vi "niRFUtil FWK Active Channel Parser.vi"(0 "Active Channel":string, 5 "String Format":string[](array[string])=[""], 7 "Number of Channels":i32=1, 11 "error in (no error)":errorcluster, 12 "Mode":enum16{"Write", "Read"}(ring)) -> (6 "Channel Index":i32[](array[numeric]), 10 "Channel Name":string, 15 "error out":errorcluster)   [LabVIEW 2015, in "niRFUtil.lvlib"]
uses:
  niRFUtil.lvlib
  <vilib>/regexp/Match Regular Expression.xnode
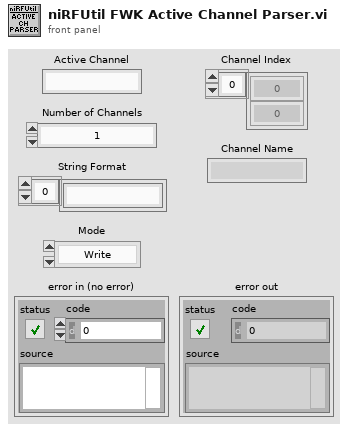
[diagram p1: front panel]
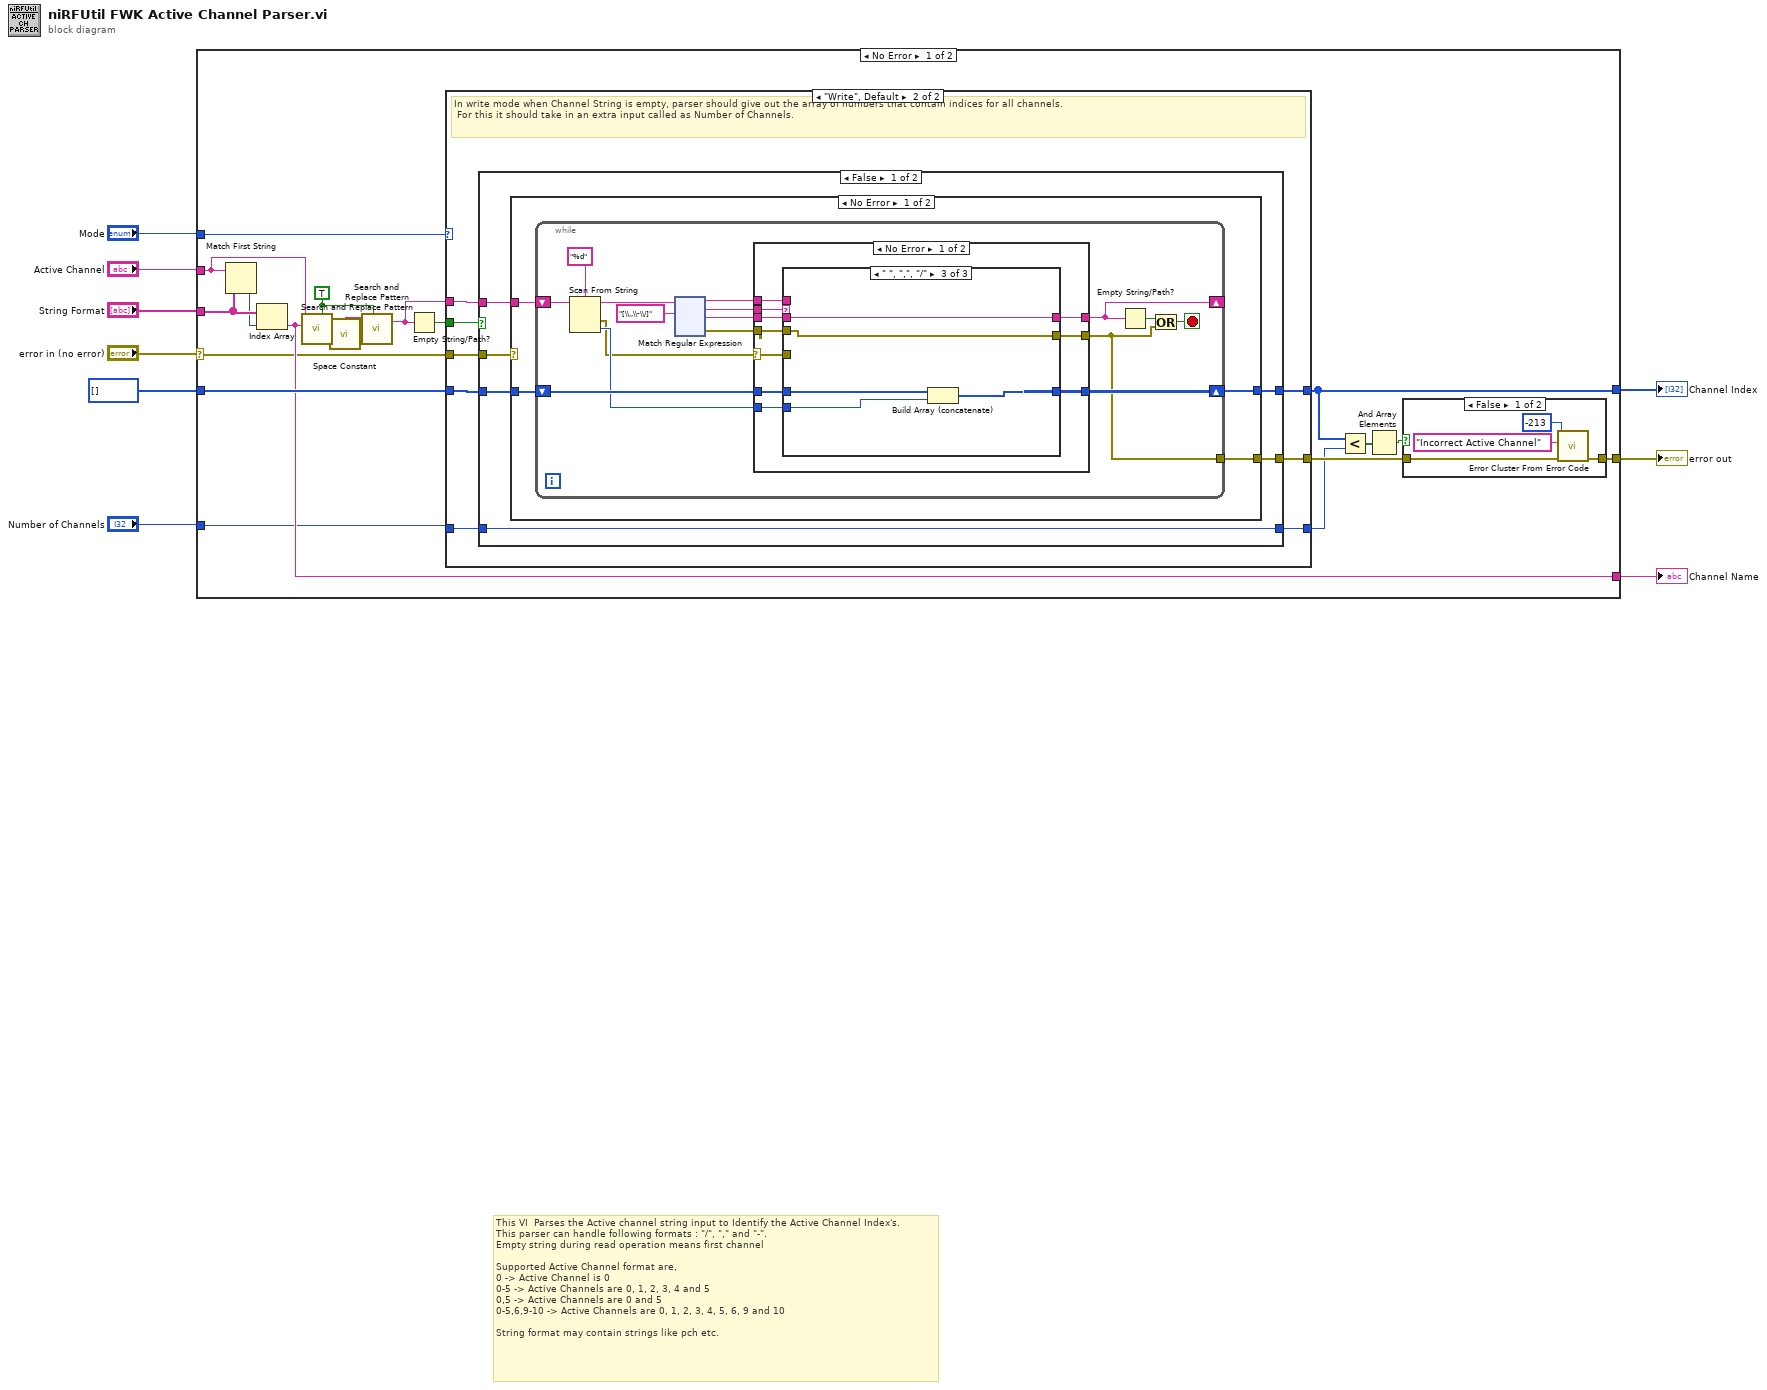
[diagram p0: block diagram]
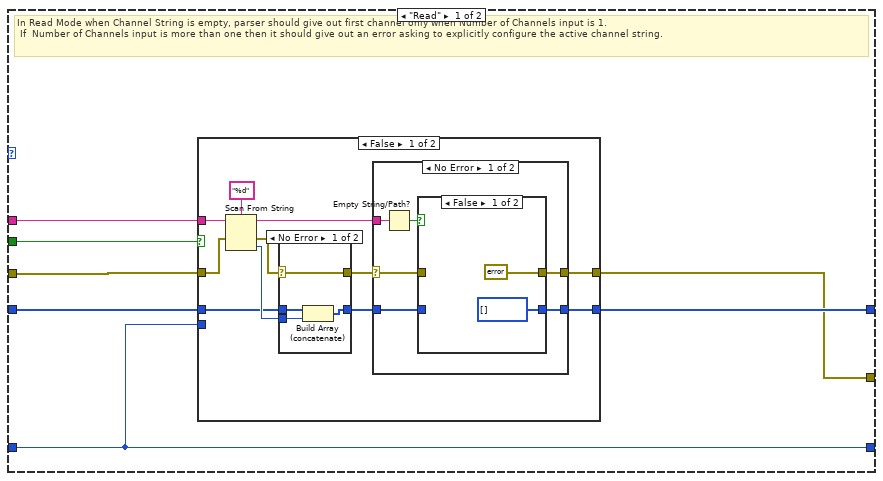
[diagram p3: hidden frame]
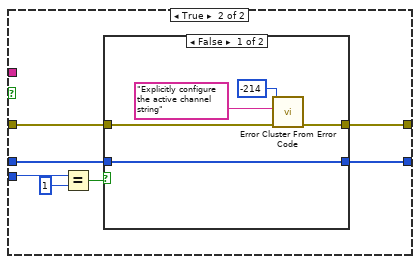
[diagram p7: hidden frame]
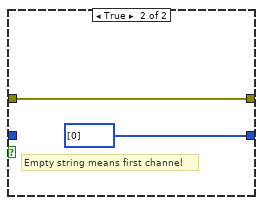
[diagram p8: hidden frame]
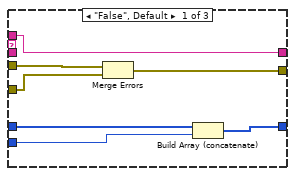
[diagram p9: hidden frame]
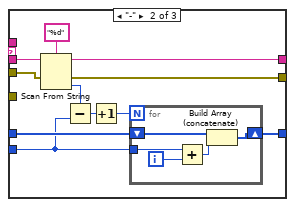
[diagram p10: hidden frame]
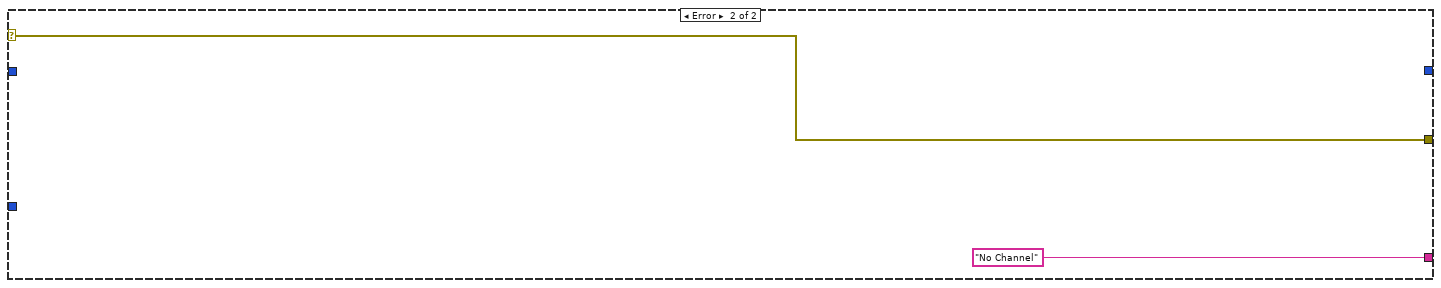
[diagram p14: hidden frame]
diagram:
  # "This VI  Parses the Active channel string input to Identify the Active Channel Index's.\nThis parser can handle following formats : \"/\", \",\" and \"-\".\nEmpty string during read operation means first channel\n\nSupported Active Channel format are,\n0 -> Active Channel is 0 \n0-5 -> Active Channels are 0, 1, 2, 3, 4 and 5\n0,5 -> Active Channels are 0 and 5\n0-5,6,9-10 -> Active Channels are 0, 1, 2, 3, 4, 5, 6, 9 and 10\n\nString format may contain strings like pch etc."
  n1 = case shown="No Error" "error in (no error)" {
    selector: "error in (no error)" -> [w22 w276]
    tunnel: i32[] [] -> [w27 _]
    tunnel: "Active Channel" -> [w24 _]
    tunnel: [w16 w276] -> w4
    tunnel: [w25 "No Channel"] -> w3
    tunnel: "Mode" -> [w23 _]
    tunnel: "String Format" -> [w21 _]
    tunnel: "Number of Channels" -> [w20 _]
    tunnel: [w15 _] -> w2
    frame No Error {
      w11 = TRUE ("replace all? (F)")
      n2 = Match First String(2:w21, 3:w24) -> (0:w14:i32)  [unwired: 1 out]
      n3 = Index Array(array=w21, index=w14) -> (element=w25:string)
      n4 = call <vilib>:"Search and Replace Pattern.vi"("string"=w24, "regular expression (\"\")"=w25, "replace all? (F)"=w11) -> ("result string"=w13:string)  [unwired: 2 in, 1 out]
      n5 = call <vilib>:"Space Constant.vi"() -> ("String"=w12:string)
      n6 = call <vilib>:"Search and Replace Pattern.vi"("string"=w13, "regular expression (\"\")"=w12, "replace all? (F)"=w11) -> ("result string"=w10:string)  [unwired: 2 in, 1 out]
      n7 = Empty String/Path?(string/path=w10) -> (empty?=w26:bool)
      n8 = case shown="\"Write\", Default" w23 {
        tunnel: w27 -> [w40 w91]
        tunnel: [w39 w90] -> w15
        tunnel: w26 -> [w38 w89]
        tunnel: [w37 w88] -> w28
        tunnel: w10 -> [w34 w87]
        tunnel: w22 -> [w36 w86]
        tunnel: w20 -> [w35 w85]
        tunnel: [w35 w84] -> w17
        frame "Read" {
          # "In Read Mode when Channel String is empty, parser should give out first channel only when Number of Channels input is 1.\n If  Number of Channels input is more than one then it should give out an error asking to explicitly configure the active channel string."
          n9 = case shown="False" w38 {
            tunnel: w40 -> [w46 w72]
            tunnel: [w51 w76] -> w39
            tunnel: w34 -> [w50 _]
            tunnel: [w42 w70] -> w37
            tunnel: w36 -> [w41 w71]
            tunnel: w35 -> [_ w75]
            frame False {
              n10 = Scan From String(format string="%d", input string=w50, error in=w41) -> (remaining string=w49:string, error out=w48:errorcluster, output 1=w47:i32)  [unwired: 2 in, 1 out]
              n11 = case shown="No Error" w48 {
                selector: w48 -> [w64 w68]
                tunnel: w47 -> [w65 _]
                tunnel: w46 -> [w67 w69]
                tunnel: [w66 w69] -> w45
                tunnel: [w64 w68] -> w43
                frame No Error {
                  n12 = Build Array (concatenate)(w67, w65) -> (w66:i32[])
                }
                frame Error {
                }
              }
              n13 = case shown="No Error" w43 {
                selector: w43 -> [w53 w62]
                tunnel: [w57 w63] -> w51
                tunnel: w49 -> [w56 _]
                tunnel: w45 -> [w55 w63]
                tunnel: [w54 w62] -> w42
                frame No Error {
                  n14 = Empty String/Path?(string/path=w56) -> (empty?=w52:bool)
                  n15 = case shown="False" w52 {
                    tunnel: [i32[] [] w61] -> w57
                    tunnel: w55 -> [_ w61]
                    tunnel: w53 -> [_ w60]
                    tunnel: [errorcluster {"status"=TRUE, "code"=-213, "source"="Incorrect Active Channel"} ("error IO") w60] -> w54
                    frame False {
                    }
                    frame True {
                    }
                  }
                }
                frame Error {
                }
              }
            }
            frame True {
              n16 = Equal?(x=w75, y=1) -> (x = y?=w73:bool)
              n17 = case shown="False" w73 {
                tunnel: [w81 i32[] [0]] -> w76
                tunnel: w72 -> [w81 _]
                tunnel: w71 -> [w77 w82]
                tunnel: [w78 w82] -> w70
                frame False {
                  n18 = call <vilib>:"Error Cluster From Error Code.vi"("error in (no error)"=w77, "error message (\"\")"="Explicitly configure the active channel string" ("error message (\"\")"), "error code (0)"=-214 ("code")) -> ("error out"=w78:errorcluster)  [unwired: 6 in]
                }
                frame True {
                  # "Empty string means first channel"
                }
              }
            }
          }
        }
        frame "Write", Default {
          # "In write mode when Channel String is empty, parser should give out the array of numbers that contain indices for all channels.\n For this it should take in an extra input called as Number of Channels."
          n19 = case shown="False" w89 {
            tunnel: w91 -> [w96 _]
            tunnel: [w97 w273] -> w90
            tunnel: w87 -> [w92 _]
            tunnel: [w94 w272] -> w88
            tunnel: w86 -> [w95 w272]
            tunnel: w85 -> [w93 w271]
            tunnel: [w93 w271] -> w84
            frame False {
              n20 = case shown="No Error" w95 {
                selector: w95 -> [_ w269]
                tunnel: [w101 w270] -> w97
                tunnel: w92 -> [w100 _]
                tunnel: w96 -> [w99 w270]
                tunnel: [w98 w269] -> w94
                frame No Error {
                  n21 = while {
                    shift-right: [w104] -> _
                    shift-left: w100 -> [w109]
                    shift-right: [w111] -> w101
                    shift-left: w99 -> [w115]
                    tunnel: [w103] -> w98
                    stop <- w112 stop-if-true
                    n22 = Scan From String(format string="%d", input string=w109) -> (remaining string=w108:string, error out=w105:errorcluster, output 1=w107:i32)  [unwired: 3 in, 1 out]
                    n23 = xnode "Match Regular Expression"("input string"=w108, "regular expression"="[\\,,\\-\\/]") -> ("before match"=w114:string, "whole match"=w117:string, "after match"=w116:string, "error out"=w106:errorcluster)  [unwired: 4 in, 1 out]
                    n24 = case shown="No Error" w105 {
                      selector: w105 -> [w118 _]
                      tunnel: w117 -> [w127 _]
                      tunnel: w116 -> [w126 w157]
                      tunnel: w115 -> [w125 w156]
                      tunnel: w114 -> [w124 _]
                      tunnel: [w123 w157] -> w104
                      tunnel: [w122 _] -> w103
                      tunnel: [w121 w156] -> w111
                      tunnel: w107 -> [w119 _]
                      tunnel: w106 -> [w120 _]
                      frame No Error {
                        n25 = case shown="\" \", \",\", \"/\"" w127 {
                          tunnel: w126 -> [_ w142 w153]
                          tunnel: [w128 w141 w153] -> w123
                          tunnel: [w132 w145 w155] -> w121
                          tunnel: w125 -> [w134 w144 w154]
                          tunnel: w124 -> [w128 _ _]
                          tunnel: [w129 w136 w151] -> w122
                          tunnel: w120 -> [w130 w135 w151]
                          tunnel: w119 -> [w133 w137 w152]
                          tunnel: w118 -> [w131 _ _]
                          frame "False", Default {
                            n26 = Merge Errors(w130, w131) -> (w129:errorcluster)
                            n27 = Build Array (concatenate)(w134, w133) -> (w132:i32[])
                          }
                          frame "-" {
                            n28 = Scan From String(format string="%d", input string=w142, error in=w135) -> (remaining string=w141:string, error out=w136:errorcluster, output 1=w139:i32)  [unwired: 2 in, 1 out]
                            n29 = Subtract(x=w139, y=w137) -> (x-y=w140:i32)
                            n30 = Increment(x=w140) -> (x+1=w138:i32)
                            n31 = for {
                              N: w138 -> [_]
                              tunnel: w137 -> [w148]
                              shift-right: [w150] -> w145
                              shift-left: w144 -> [w149]
                              i -> [w146]
                              n32 = Add(x=w148, y=w146) -> (x+y=w147:i32)
                              n33 = Build Array (concatenate)(w149, w147) -> (w150:i32[])
                            }
                          }
                          frame " ", ",", "/" {
                            n34 = Build Array (concatenate)(w154, w152) -> (w155:i32[])
                          }
                        }
                      }
                      frame Error {
                      }
                    }
                    n35 = Empty String/Path?(string/path=w104) -> (empty?=w113:bool)
                    n36 = Or(x=w113, y=w103) -> (x .or. y?=w112:bool)
                  }
                }
                frame Error {
                }
              }
            }
            frame True {
              n37 = for {
                N: w271 -> [_]
                tunnel: [w274] -> w273 mode=indexing
                i -> [w274]
              }
            }
          }
        }
      }
      n38 = Less?(x=w15, y=w17) -> (x < y?=w19:bool[])
      n39 = And Array Elements(Boolean array=w19) -> (logical AND=w18:bool)
      n40 = case shown="False" w18 {
        tunnel: w28 -> [w30 w33]
        tunnel: [w29 w33] -> w16
        frame False {
          n41 = call <vilib>:"Error Cluster From Error Code.vi"("error in (no error)"=w30, "error message (\"\")"="Incorrect Active Channel" ("error message (\"\")"), "error code (0)"=-213 ("code")) -> ("error out"=w29:errorcluster)  [unwired: 6 in]
        }
        frame True {
        }
      }
    }
    frame Error {
    }
  }
  "Channel Index" <- w2
  "Channel Name" <- w3
  "error out" <- w4
